vi "OpenCvGlobals.vi"() -> ()   [LabVIEW 2012]
panel:
  in  "initialized":bool
  out "opencv semaphore":T1
  out "frameNumberBright":i32
  out "rotBright":dbl
  out "centerYBright":dbl
  out "centerXBright":dbl
  out "found fly":i32
  out "ySize":i32
  out "xSize":i32
  out "error":errorcluster
  in  "isDebug":bool
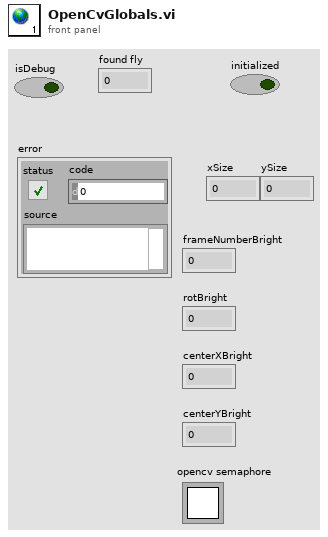
[diagram p1: front panel]
types:
  T1 = typedef "Semaphore RefNum" = refnum<k1>
diagram:
